vi "fitsErrText.vi"(11 "status":i32) -> (3 "message":string)   [LabVIEW 2019]
doc: "Return a descriptive text string (30 char max.) corresponding to a CFITSIO error status code. A wrapper for fits_get_errstatus()"
uses:
  F:/INO340/OSL/Beta Release/V0-3-1/PTC_src_V0-3-1/Common/lib/libfits.dll
panel:
  out "return type":i32
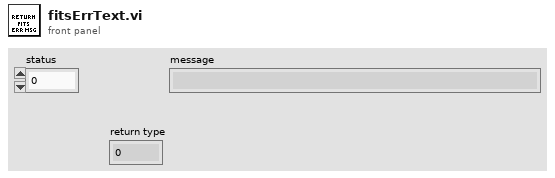
[diagram p1: front panel]
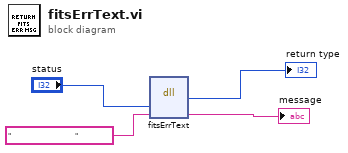
[diagram p0: block diagram]
diagram:
  n1 = dll-call lib="F:/INO340/OSL/Beta Release/V0-3-1/PTC_src_V0-3-1/Common/lib/libfits.dll" fn="fitsErrText"("status"="status", "message"="                                ") -> ("return type"=→"return type":i32, "message"=→"message":string)  [unwired: 4 in, 2 out]
